vi "GetEventListings.vi"(8 "error in (no error)":errorcluster, 11 "Append to URL":string) -> (0 "error out":errorcluster, 1 "eventCount":dbl, 3 "output cluster":T1)   [LabVIEW 2014, in "FIRST Events API.lvlib"]
uses:
  FIRST Events API.lvlib
  FRC Event Listings.ctl
  Backend/source/VI Source/FRCts20_Backend_API/FRCts20_Backend_API_EventRoot.ctl
  FRC API Selector.ctl
  Backend/source/VI Source/FRCts20_Backend_API/FRCts20_Backend_API.lvlib
panel:
  out "value":T2
  out "body":string
  out "headers":string
  out "Generated URL":string
  # "returns all FRC official district and regional events in a particular season"
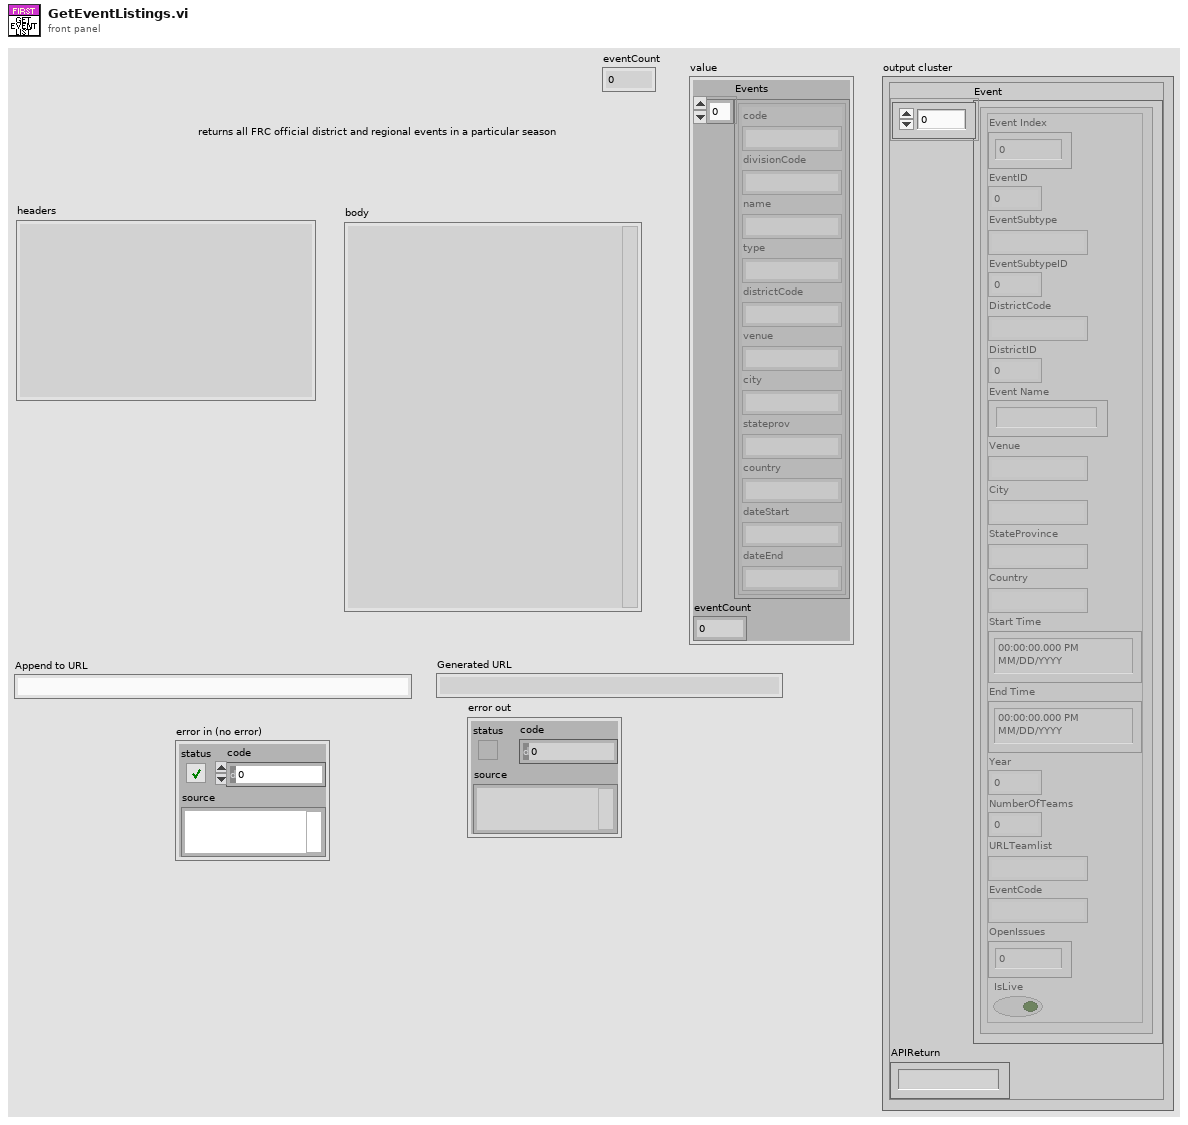
[diagram p1: front panel]
types:
  T1 = typedef "FRCts20_Backend_API.lvlib/FRCts20_Backend_API_EventRoot.ctl" = cluster{"Event":cluster{"Event Index":u32, "EventID":u32, "EventSubtype":string, "EventSubtypeID":u32, "DistrictCode":string, "DistrictID":u32, "Event Name":string, "Venue":string, "City":string, "StateProvince":string, "Country":string, "Start Time":timestamp, "End Time":timestamp, "Year":u32, "NumberOfTeams":u32, "URLTeamlist":string, "EventCode":string, "OpenIssues":u8, "IsLive":bool}[], "APIReturn":string}
  T2 = typedef "FIRST Events API.lvlib/FRC Event Listings.ctl" = cluster{"Events":cluster{"code":string, "divisionCode":string, "name":string, "type":string, "districtCode":string, "venue":string, "city":string, "stateprov":string, "country":string, "dateStart":string, "dateEnd":string}[], "eventCount":dbl}
  T3 = typedef "FIRST Events API.lvlib/FRC API Selector.ctl" = enum16{"GetEventAllianceSelection", "Ancillary", "GetTeamListings", "GetSchedule", "GetEventListings"}
  T4 = cluster{"code":string, "divisionCode":string, "name":string, "type":string, "districtCode":string, "venue":string, "city":string, "stateprov":string, "country":string, "dateStart":string, "dateEnd":string}[]
  T5 = cluster{"Event Index":u32, "EventID":u32, "EventSubtype":string, "EventSubtypeID":u32, "DistrictCode":string, "DistrictID":u32, "Event Name":string, "Venue":string, "City":string, "StateProvince":string, "Country":string, "Start Time":timestamp, "End Time":timestamp, "Year":u32, "NumberOfTeams":u32, "URLTeamlist":string, "EventCode":string, "OpenIssues":u8, "IsLive":bool}
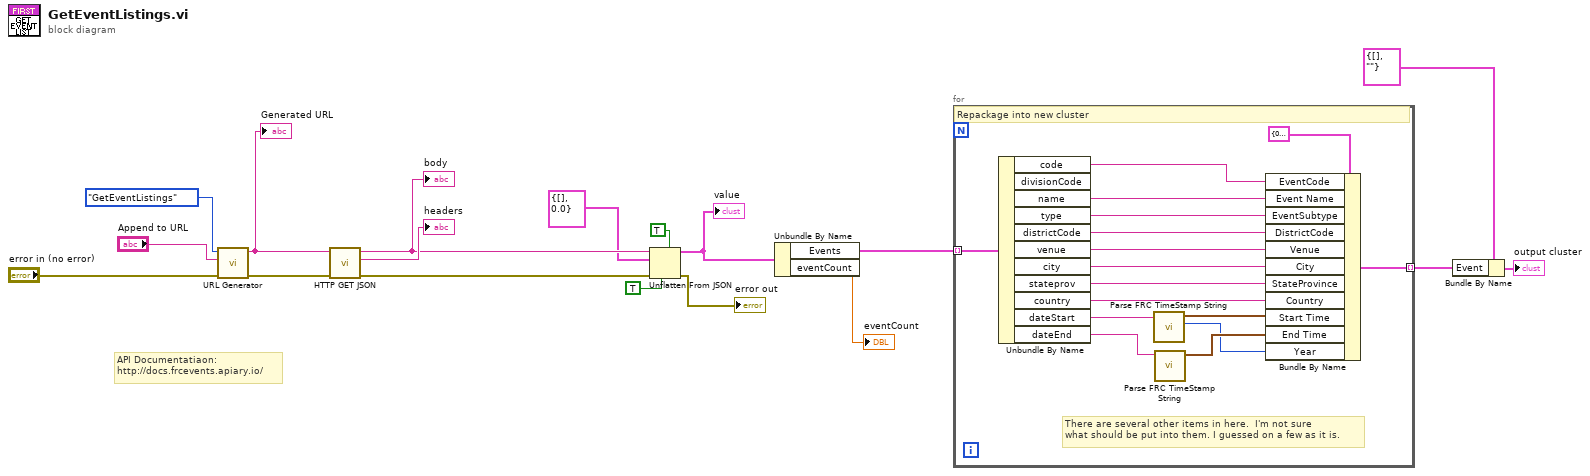
[diagram p0: block diagram]
diagram:
  # "API Documentatiaon:\nhttp://docs.frcevents.apiary.io/"
  n1 = call "URL Generator.vi"("error in (no error)"="error in (no error)", "Append URL"="Append to URL", "API Command"=FRC_API_Selector."GetEventListings") -> ("error out"=w13:errorcluster, "Generated URL"=w16:string)  [unwired: 7 in]
  "Generated URL" <- w16
  n2 = call "HTTP GET JSON.vi"("error in (no error)"=w13, "Generated URL"=w16) -> ("error out"=w11:errorcluster, "headers"=→"headers":string, "body"=w12:string)  [unwired: 7 in]
  "body" <- w12
  n3 = Unflatten From JSON(enable LabVIEW extensions? (T)=TRUE, JSON string=w12, type and defaults=T2 {"Events"=[], "eventCount"=0.0} ("Events"), default null elements? (F)=TRUE, error in (no error)=w11) -> (value=w7:T2, error out=→"error out":errorcluster)  [unwired: 2 in]
  "value" <- w7
  n4 = Unbundle By Name(w7) -> ("Events"=w6:T4, "eventCount"=→"eventCount":dbl)
  n5 = for {
    tunnel: w6 -> [w34] mode=indexing
    tunnel: [w20] -> w4 mode=indexing
    # "There are several other items in here.  I'm not sure\nwhat should be put into them. I guessed on a few as it is."
    # "Repackage into new cluster"
    n6 = Unbundle By Name(w34) -> ("code"=w21:string, "name"=w22:string, "type"=w23:string, "districtCode"=w24:string, "venue"=w33:string, "city"=w32:string, "stateprov"=w31:string, "country"=w30:string, "dateStart"=w29:string, "dateEnd"=w27:string)  [unwired: 1 out]
    n7 = call "Parse FRC TimeStamp String.vi"("date/time string"=w29) -> ("year"=w25:i32, "Resulting Time Stamp"=w28:timestamp)  [unwired: 9 in]
    n8 = call "Parse FRC TimeStamp String.vi"("date/time string"=w27) -> ("Resulting Time Stamp"=w26:timestamp)  [unwired: 9 in, 1 out]
    n9 = Bundle By Name(cluster=T5 {"Event Index"=0, "EventID"=0, "EventSubtype"="", "EventSubtypeID"=0, "DistrictCode"="", "DistrictID"=0, "Event Name"="", "Venue"="", "City"="", "StateProvince"="", "Country"="", "Start Time"=timestamp(0 s since 1904-01-01), "End Time"=timestamp(0 s since 1904-01-01), "Year"=0, "NumberOfTeams"=0, "URLTeamlist"="", "EventCode"="", "OpenIssues"=0, "IsLive"=FALSE} ("Cluster"), "EventCode"=w21, "Event Name"=w22, "EventSubtype"=w23, "DistrictCode"=w24, "Venue"=w33, "City"=w32, "StateProvince"=w31, "Country"=w30, "Start Time"=w28, "End Time"=w26, "Year"=w25) -> (w20:T5)
  }
  n10 = Bundle By Name(cluster=T1 {"Event"=[], "APIReturn"=""} ("Events"), "Event"=w4) -> (→"output cluster":T1)
